vi "set Enable Debugging.vi"(10 "Enable Debugging":bool, 11 "Actor in":refnum<class "Actor.lvclass">) -> (3 "Actor out":refnum<class "Actor.lvclass">)   [LabVIEW 2015, in "Actor.lvclass"]
uses:
  Actor.lvclass
  Actor.lvclass/Actor.ctl
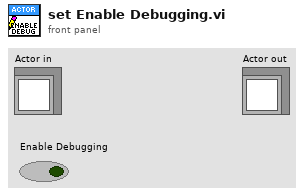
[diagram p1: front panel]
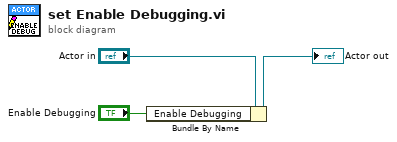
[diagram p0: block diagram]
diagram:
  n1 = Bundle By Name(cluster="Actor in", "Enable Debugging"="Enable Debugging") -> (→"Actor out":refnum<class "Actor.lvclass">)
